vi "Open Example.vi"   [LabVIEW 2021, in "Async Methods Actor.lvlib"]
uses:
  Async Methods Actor.lvlib
panel:
  # "Run this VI to open the the \"Async Methods Actor Example\""
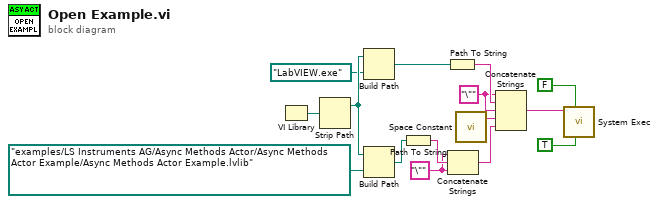
[diagram p0: block diagram]
diagram:
  w7 = "\""
  w9 = "\""
  n1 = VI Library() -> (path=w15:path)
  n2 = Strip Path(path=w15) -> (stripped path=w13:path)  [unwired: 1 out]
  n3 = Build Path(base path=w13, name or relative path=path "LabVIEW.exe") -> (appended path=w11:path)
  n4 = Build Path(base path=w13, name or relative path=path "examples/LS Instruments AG/Async Methods Actor/Async Methods Actor Example/Async Methods Actor Example.lvlib") -> (appended path=w6:path)
  n5 = Path To String(path=w6) -> (string=w8:string)
  n6 = Path To String(path=w11) -> (string=w10:string)
  n7 = Concatenate Strings(w7, w8, w7) -> (w4:string)
  n8 = call <vilib>:"Space Constant.vi"() -> ("String"=w5:string)
  n9 = Concatenate Strings(w9, w10, w9, w5, w4) -> (w3:string)
  n10 = call <vilib>:"System Exec.vi"("run minimized? (F)"=TRUE, "wait until completion? (T)"=FALSE, "command line"=w3) -> ()  [unwired: 5 in, 4 out]
